vi "Actor Core.vi"(8 "error in":errorcluster, 11 "Nested in":refnum<class "MSS Remote Actor.lvclass">) -> (0 "error out":errorcluster, 3 "Actor out":refnum<class "Actor.lvclass">)   [LabVIEW 2023, in "MSS Remote Actor.lvlib" / "MSS Remote Actor.lvclass"]
doc: "(<B>Filename</B>: Actor Framework.lvlib:Actor.lvclass:Actor Core.vi)\n\nReceives messages to the actor, reacts to them, and initiates any error handling that may shut the actor down.\n\nDescendant classes may override this VI to append parallel tasks for the actor to complete while it handles messages. Overrides use the Call Parent Method node."
uses:
  MSS Remote Actor.lvclass
  MSS Remote Actor.lvclass/MSS Remote Actor.ctl
  <vilib>/ActorFramework/Actor/Actor.lvclass
  <vilib>/ActorFramework/Stop Msg/Stop Msg.lvclass
  HAL GOOP4/Measure and Stimulus Subsystems/Measure and Stimulus Subsystems.lvclass
panel:
  out "Intrs Configs":T1
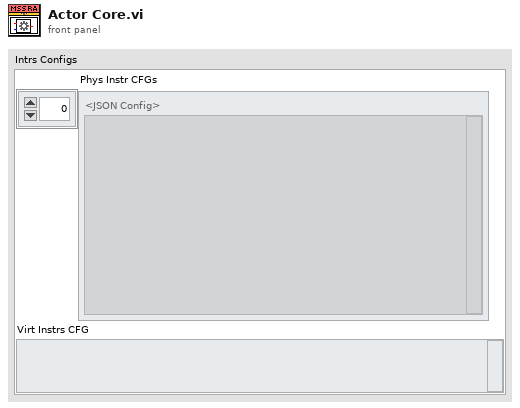
[diagram p1: front panel]
types:
  T1 = cluster{"Phys Instr CFGs":string[], "Virt Instrs CFG":string}
  T2 = cluster{"Stop":refnum<user-event>, "Intrs Configs":refnum<user-event>}
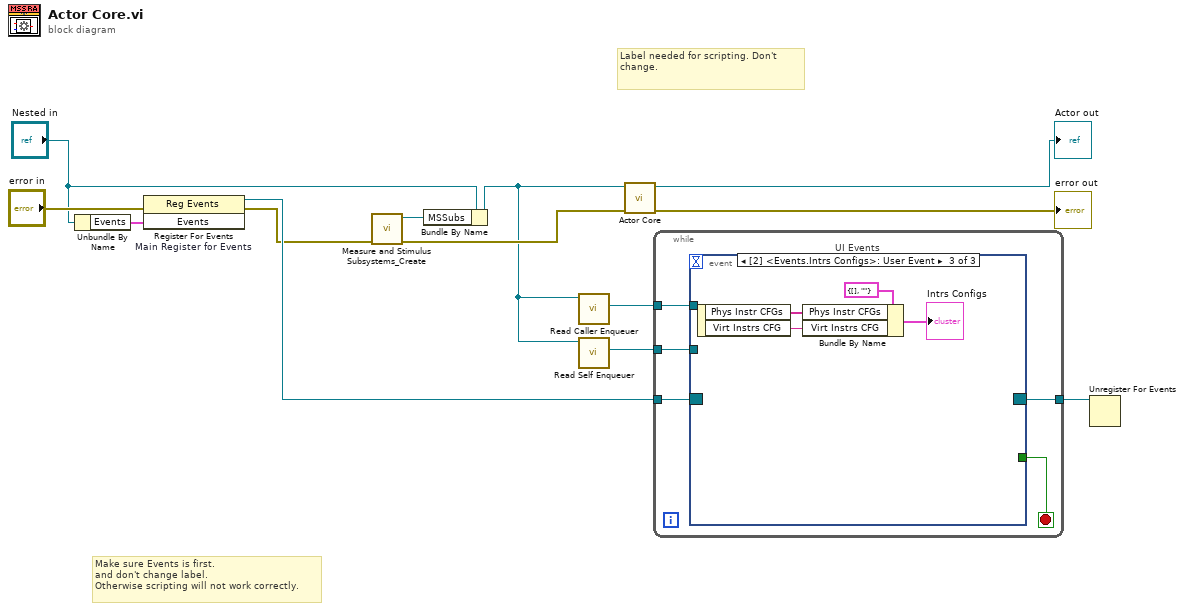
[diagram p0: block diagram]
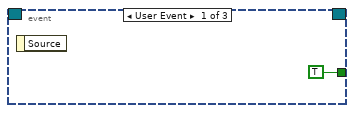
[diagram p2: hidden frame]
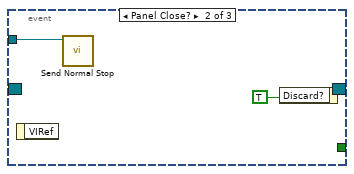
[diagram p3: hidden frame]
diagram:
  # "Label needed for scripting. Don't change."
  # "Make sure Events is first.\nand don't change label.\nOtherwise scripting will not work correctly."
  n1 = Unbundle By Name("Nested in") -> ("Events"=w10:T2)
  n2 = register-events "Main Register for Events"(error in="error in", w10) -> (reference out=w11:refnum<event-registration>, error out=w6:errorcluster)  [unwired: 1 in]
  n3 = call "Measure and Stimulus Subsystems_Create.vi"("Error In"=w6) -> ("Error Out"=w5:errorcluster, "reference out"=w4:refnum<class "Measure and Stimulus Subsystems.lvclass">)  [unwired: 9 in]
  n4 = Bundle By Name(cluster="Nested in", "MSSubs"=w4) -> (w2:refnum<class "MSS Remote Actor.lvclass">)
  n5 = call <vilib>:"Read Caller Enqueuer.vi"("Actor"=w2) -> ("Caller Enqueuer"=w1:refnum<class "Message Enqueuer.lvclass">)  [unwired: 10 in]
  n6 = call <vilib>:"Read Self Enqueuer.vi"("Actor"=w2) -> ("Self Enqueuer"=w8:refnum<class "Message Enqueuer.lvclass">)  [unwired: 10 in]
  n7 = call-parent "Actor Core.vi"("error in"=w5, "Actor in"=w2) -> ("error out"=→"error out":errorcluster, "Actor out"=→"Actor out":refnum<class "Actor.lvclass">)  [unwired: 8 in]
  n8 = while {
    tunnel: w11 -> [w18]
    tunnel: [w16] -> w9
    tunnel: w8 -> [w15]
    tunnel: w1 -> [w14]
    stop <- w17 stop-if-true
    n9 = event "UI Events" shown="[2] <Events.Intrs Configs>: User Event" {
      selector: w18 -> [_ _ _]
      dyn-events: [_ _ _] -> w16
      timeout: _ -> [_ _ _]
      tunnel: [TRUE _ _] -> w17
      tunnel: w15 -> [_ w20 _]
      tunnel: w14 -> [_ _ _]
      event User Event {
        n10 = event-data() -> ()  [unwired: 1 in, 1 out]
      }
      event Panel Close? {
        n11 = event-data() -> ()  [unwired: 1 in, 1 out]
        n12 = call <vilib>:"Send Normal Stop.vi"("Message Enqueuer"=w20) -> ()  [unwired: 10 in, 1 out]
        n13 = event-data("Discard?"=TRUE) -> ()  [unwired: 1 in, 1 out]
      }
      event User Event {
        n14 = event-data() -> ("Phys Instr CFGs"=w24:string[], "Virt Instrs CFG"=w23:string)  [unwired: 1 in]
        n15 = Bundle By Name(cluster=T1 {"Phys Instr CFGs"=[], "Virt Instrs CFG"=""} ("Intrs Configs"), "Phys Instr CFGs"=w24, "Virt Instrs CFG"=w23) -> (→"Intrs Configs":T1)
      }
    }
  }
  n16 = Unregister For Events(event registration refnum=w9) -> ()  [unwired: 1 in, 1 out]
